vi "testEmbeddedXML.vi"(8 "error in (no error)":errorcluster, 11 "reference in":refnum<class "EasyXMLTest.lvclass">) -> (0 "error out":errorcluster, 3 "reference in":refnum<class "EasyXMLTest.lvclass">)   [LabVIEW 2013, in "EasyXMLTest.lvclass"]
uses:
  EasyXMLTest.lvclass
  <vilib>/addons/_JKI Toolkits/VI Tester/TestCase.llb/TestCase.lvclass
panel:
  out "Produced Data":cluster{"XMLString":string}
  out "Generated XML String":string
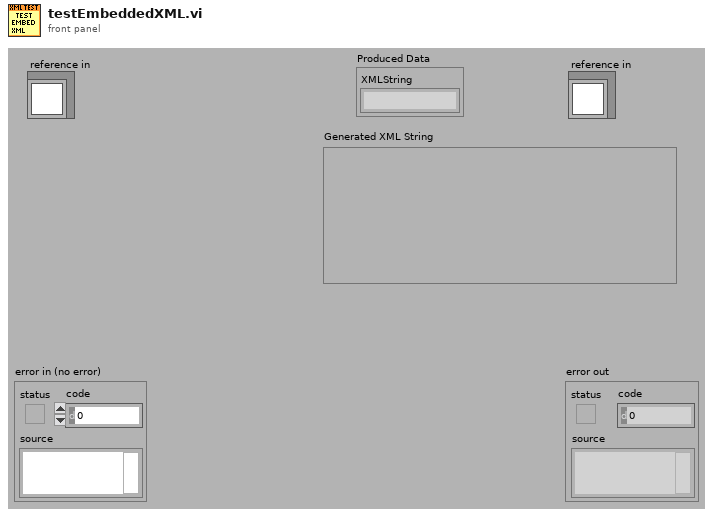
[diagram p1: front panel]
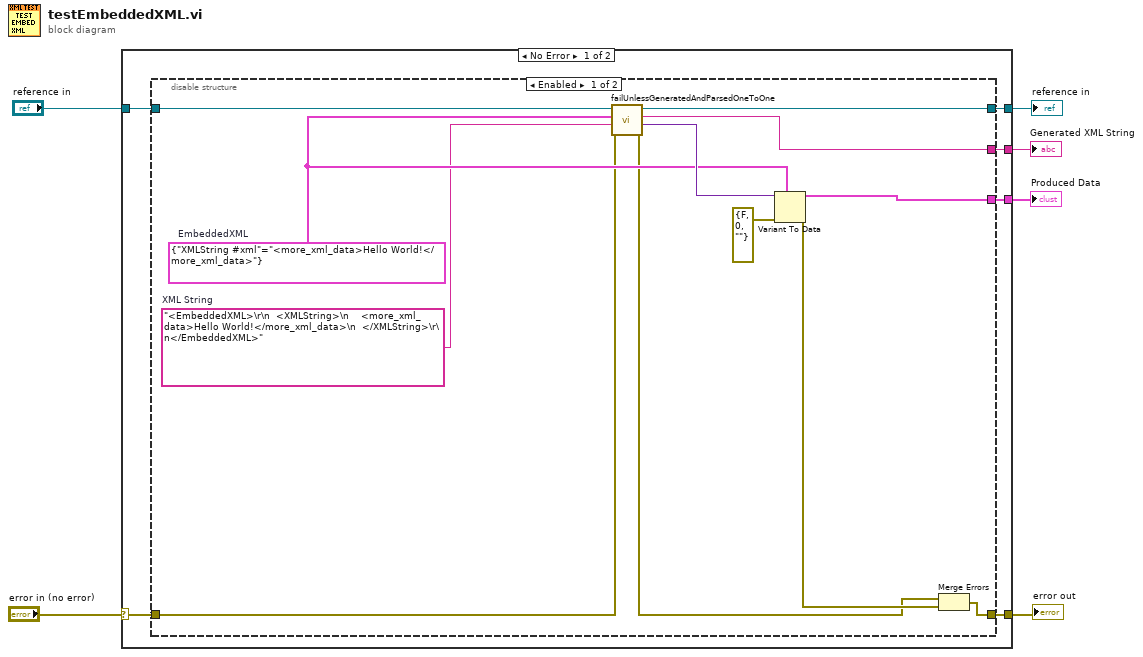
[diagram p0: block diagram]
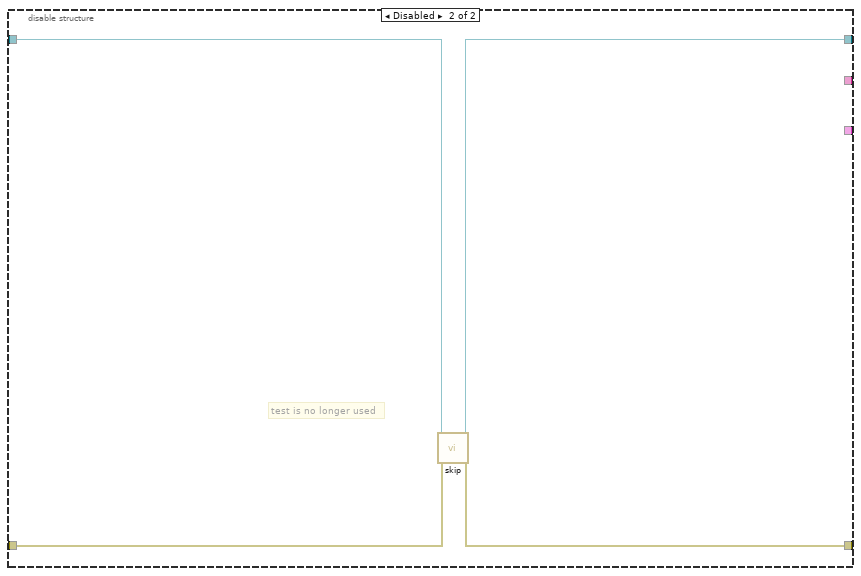
[diagram p2: hidden frame]
diagram:
  n1 = case shown="No Error" "error in (no error)" {
    selector: "error in (no error)" -> [w7 w30]
    tunnel: [w12 w30] -> w5
    tunnel: [w9 w29] -> w3
    tunnel: "reference in" -> [w10 w29]
    tunnel: [w8 _] -> w2
    tunnel: [w11 _] -> w1
    frame No Error {
      n2 = disable-structure shown="Enabled" {
        disable-tunnel: [w23 w25] -> w12
        disable-tunnel: [w22 _] -> w11
        disable-tunnel: w10 -> [w20 w28]
        disable-tunnel: [w19 w27] -> w9
        disable-tunnel: [w17 _] -> w8
        disable-tunnel: w7 -> [w14 w26]
        frame Enabled {
          w15 = "<EmbeddedXML>\r\n  <XMLString>\n    <more_xml_data>Hello World!</more_xml_data>\n  </XMLString>\r\n</EmbeddedXML>"  # XML String
          w16 = cluster{"XMLString #xml":string} {"XMLString #xml"="<more_xml_data>Hello World!</more_xml_data>"}  # EmbeddedXML
          n3 = call "failUnlessGeneratedAndParsedOneToOne.vi"("error in"=w14, "XML String"=w15, "Data"=w16, "EasyXMLTest in"=w20) -> ("error out"=w13:errorcluster, "Produced Data"=w18:variant, "Generated XML String"=w17:string, "EasyXMLTest out"=w19:refnum<class "EasyXMLTest.lvclass">)  [unwired: 4 in]
          n4 = Variant To Data(error in=errorcluster {"status"=FALSE, "code"=0, "source"=""}, type=w16, Variant=w18) -> (data=w22:cluster{"XMLString #xml":string}, error out=w24:errorcluster)
          n5 = Merge Errors(w13, w24) -> (w23:errorcluster)
        }
        frame Disabled {
          # "test is no longer used"
          n6 = call <vilib>:"skip.vi"("error in (no error)"=w26, "TestCase in"=w28) -> ("error out"=w25:errorcluster, "TestCase out"=w27:refnum<class "EasyXMLTest.lvclass">)  [unwired: 8 in]
        }
      }
    }
    frame Error {
    }
  }
  "error out" <- w5
  "reference in" <- w3
  "Generated XML String" <- w2
  "Produced Data" <- w1
